vi "find PUT center.vi"   [LabVIEW 2021, in "Test VIs.lvclass"]
uses:
  Test VIs/Test VIs.lvclass
  Classes/Workspace/Pick Up Tool Area/Pick Up Tool Fixture.lvclass
  Classes/Routine/Pick and Place/Pick and Place.lvclass
  Classes/Routine/Pick and Place/Pick and Place Type.ctl
  Classes/Assembly/Database Entry/Database Entry.lvclass
  Classes/Routine/Pick and Place/Pick and Place.lvclass/Pick and Place.ctl
  Classes/Routine/Pick and Place/Write Pick and Place Type.vi
  Classes/Controller/Controller.lvclass
types:
  T1 = typedef "Pick and Place.lvclass/Pick and Place Type.ctl" = enum16{"Primary Pick Up", "Secondary Pick Up", "Put Down All", "Pick Up All", "Put Down Secondary"}
  T2 = typedef "Controller.lvclass/Controllers.ctl" = cluster{"I-O.lvclass":refnum<class "I-O.lvclass">, "Gantry":refnum<k24>, "Dispenser":refnum<visa-resource-name>}
  T3 = typedef "Fixture.lvclass/Workspace.ctl" = cluster{"XYZTheta":dbl[], "Workspace Valve":i32, "Workspace Sensor":i32, "Tray Number":i32, "Position":i32, "Assembly Type":string, "Numeric":dbl, "First Pos":i32}
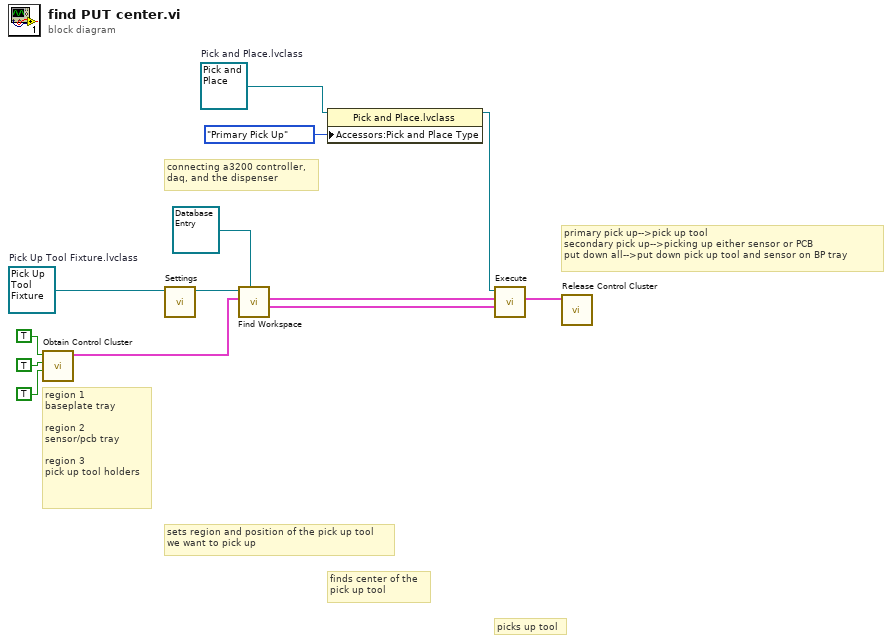
[diagram p0: block diagram]
diagram:
  w10 = refnum<class "Pick and Place.lvclass"> refnum  # Pick and Place.lvclass
  w12 = refnum<class "Pick Up Tool Fixture.lvclass"> refnum  # Pick Up Tool Fixture.lvclass
  # "primary pick up-->pick up tool\nsecondary pick up-->picking up either sensor or PCB\nput down all-->put down pick up tool and sensor on BP tray"
  # "picks up tool"
  # "finds center of the \npick up tool"
  # "connecting a3200 controller,\ndaq, and the dispenser"
  # "region 1\nbaseplate tray\n\nregion 2 \nsensor/pcb tray \n\nregion 3 \npick up tool holders"
  # "sets region and position of the pick up tool\nwe want to pick up"
  n1 = call "Obtain Control Cluster.vi"("I/O"=TRUE, "Dispense"=TRUE, "Motion"=TRUE) -> ("Control Out"=w13:T2)  [unwired: 7 in, 1 out]
  n2 = call-dynamic "Settings.vi"("Workspace in"=w12) -> ("Workspace out"=w11:refnum<class "Pick Up Tool Fixture.lvclass">)  [unwired: 9 in, 1 out]
  n3 = call-dynamic "Find Workspace.vi"("Database Entry in"=refnum<class "Database Entry.lvclass"> refnum, "Control In"=w13, "Workspace In"=w11) -> ("Workspace Out"=w7:T3, "Control Out"=w3:T2)  [unwired: 4 in, 3 out]
  n4 = property class="Pick and Place.lvclass"(reference=w10, "Accessors:Pick and Place Type"=Pick_and_Place_Type."Primary Pick Up" ("Pick and Place Type")) -> (reference out=w8:refnum<class "Pick and Place.lvclass">)  [unwired: 1 in, 1 out]
  n5 = call-dynamic "Execute.vi"("Workspace"=w7, "Cluster"=w3, "Pick and Place in"=w8) -> ("Control Out"=w2:T2)  [unwired: 6 in, 2 out]
  n6 = call "Release Control Cluster.vi"("output cluster"=w2) -> ()  [unwired: 11 in]
